vi "Y5140_ON_OFF.vi"(8 "error in (no error)":errorcluster caption="错误输入（无错误）", 9 "Turn ON/OFF":bool, 11 "MyIndex":u8) -> (0 "error out":errorcluster caption="错误输出", 1 "T/F":bool)   [LabVIEW 2015]
uses:
  <vilib>/Instr/_visa.llb/VISA Configure Serial Port (Instr).vi
panel:
  out "VISA":refnum<visa-resource-name> caption="VISA资源名称输出"
  out "Rx":string
  out "Tx":string
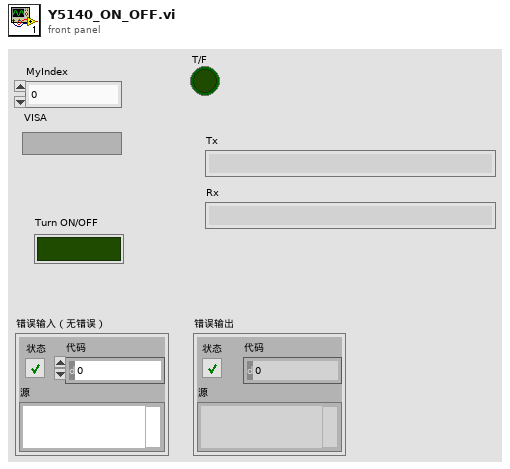
[diagram p1: front panel]
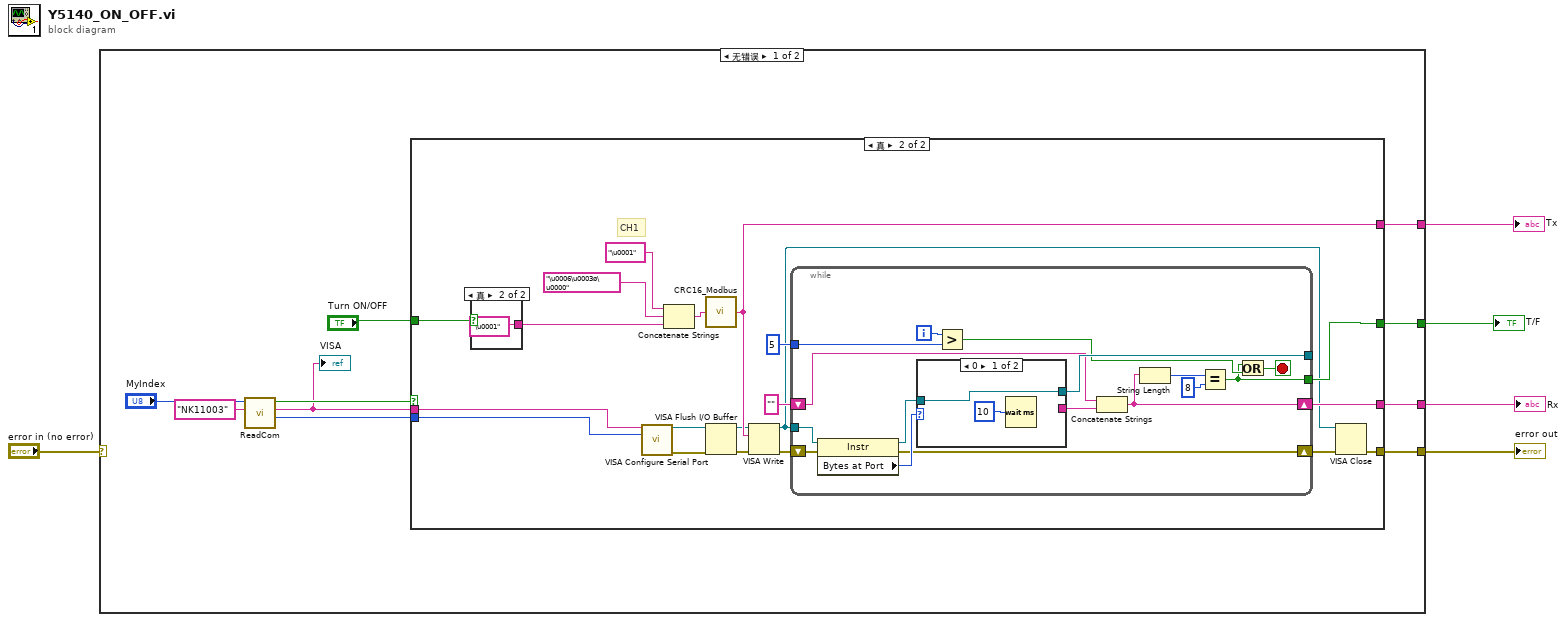
[diagram p0: block diagram]
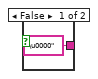
[diagram p3: hidden frame]
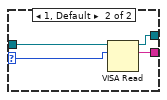
[diagram p4: hidden frame]
diagram:
  n1 = case shown="无错误" "error in (no error)" {
    selector: "error in (no error)" -> [_ w60]
    tunnel: [w15 w60] -> w5
    tunnel: [w14 _] -> w4
    tunnel: [w13 _] -> w3
    tunnel: [w11 _] -> w2
    frame No Error {
      n2 = call "ReadCom.vi"("仪器名称"="NK11003", "MyIndex"="MyIndex") -> ("Baudrate"=w6:i32, "COM"=w7:string, "OK?"=w8:bool)  [unwired: 7 in]
      "VISA" <- w7
      n3 = case shown="真" w8 {
        tunnel: [_ w17] -> w15
        tunnel: [_ w34] -> w14
        tunnel: [_ w33] -> w13
        tunnel: "Turn ON/OFF" -> [_ w24]
        tunnel: [_ w22] -> w11
        tunnel: w7 -> [_ w19]
        tunnel: w6 -> [_ w18]
        frame False {
        }
        frame True {
          # "CH1"
          n4 = case shown="真" w24 {
            tunnel: ["\u0000" "\u0001"] -> w23
            frame False {
            }
            frame True {
            }
          }
          n5 = call-poly "VISA Configure Serial Port"("VISA resource name"=w19, "baud rate (9600)"=w18) -> ("VISA resource name out"=w20:refnum<visa-resource-name>, "error out"=w21:errorcluster)  [unwired: 12 in]
          n6 = Concatenate Strings("\u0001", "\u0006\u0003ø\u0000", w23) -> (w25:string)
          n7 = call "CRC16_Modbus.vi"("需要校验的数据"=w25) -> ("String+CRC16"=w34:string)
          n8 = VISA Flush I/O Buffer(VISA resource name=w20, error in (no error)=w21) -> (VISA resource name out=w31:refnum<visa-resource-name>, error out=w30:errorcluster)  [unwired: 1 in]
          n9 = VISA Write(VISA resource name=w31, write buffer=w34, error in (no error)=w30) -> (VISA resource name out=w16:refnum<visa-resource-name>, error out=w29:errorcluster)  [unwired: 1 out]
          n10 = while {
            tunnel: w16 -> [w53]
            tunnel: [w50] -> _
            shift-right: [w41] -> w33
            shift-left: "" -> [w48]
            tunnel: 5 ("y") -> [w46]
            tunnel: [w38] -> w22
            shift-right: [w42] -> w35
            shift-left: w29 -> [w43]
            i -> [w47]
            stop <- w44 stop-if-true
            n11 = property class="Instr"(reference=w53, error in=w43) -> (reference out=w51:refnum<visa-resource-name>, error out=w42:errorcluster, "Bytes at Port"=w52:u32)
            n12 = case shown="0" w52 {
              selector: w52 -> [_ w58]
              tunnel: w51 -> [w55 w59]
              tunnel: [w55 w57] -> w50
              tunnel: [_ w56] -> w49
              frame 0 {
                n13 = Wait (ms)(milliseconds to wait=u32 10 ("等待时间（毫秒）")) -> ()  [unwired: 1 out]
              }
              frame 1, Default {
                n14 = VISA Read(VISA resource name=w59, byte count=w58) -> (VISA resource name out=w57:refnum<visa-resource-name>, read buffer=w56:string)  [unwired: 1 in, 2 out]
              }
            }
            n15 = Greater?(x=w47, y=w46) -> (0:w45:bool)
            n16 = Concatenate Strings(w48, w49) -> (w41:string)
            n17 = String Length(string=w41) -> (length=w40:i32)
            n18 = Equal?(x=w40, y=8) -> (x = y?=w38:bool)
            n19 = Or(x=w38, y=w45) -> (x .or. y?=w44:bool)
          }
          n20 = VISA Close(VISA resource name=w16, error in (no error)=w35) -> (error out=w17:errorcluster)
        }
      }
    }
    frame Error {
    }
  }
  "error out" <- w5
  "Tx" <- w4
  "Rx" <- w3
  "T/F" <- w2
